vi "Bundle Zero PAS Values.vi"(7 "pasValuesByFilter In":refnum<k24>[](array[refnum]), 8 "error in (no error)":errorcluster, 10 "Results":T2[](array[typedef]), 11 "Filter Sequences":T1[](array[typedef])) -> (0 "error out":errorcluster, 1 "pasValuesByFilter Out":refnum<k24>[](array[refnum]), 4 "Filter Sequences Out":T1[](array[typedef]))   [LabVIEW 2015]
uses:
  Controls/Test Info.ctl
  Controls/Filter Sequence.ctl
  C:/Distributed/CalFlex.dll
  CalFlex.dll
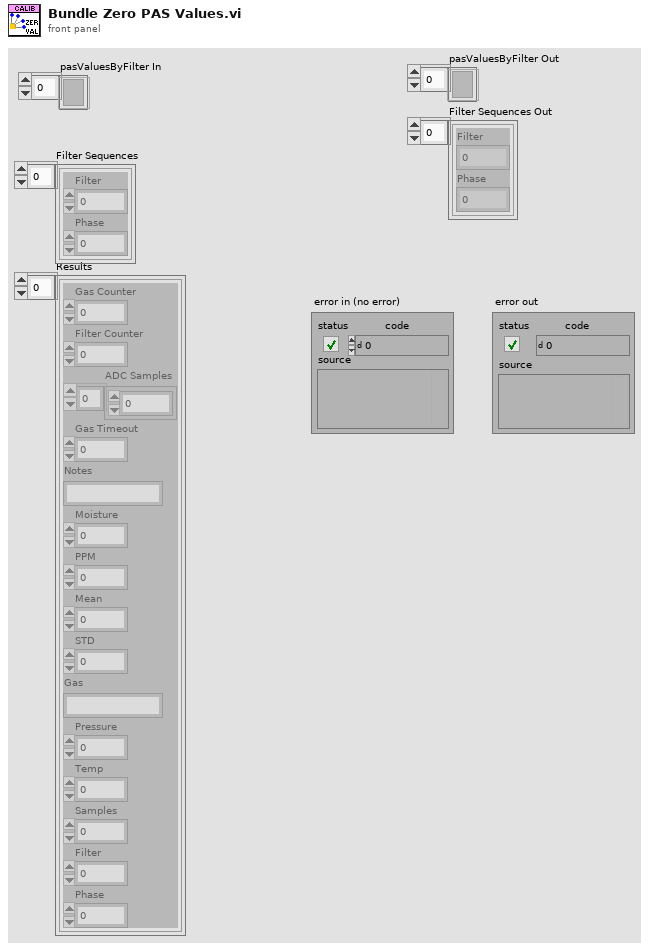
[diagram p1: front panel]
types:
  T1 = typedef "Filter Sequence.ctl" = cluster{"Filter":u8, "Phase":dbl}
  T2 = typedef "Test Info.ctl" = cluster{"Gas Counter":u16, "Filter Counter":u16, "ADC Samples":dbl[], "Gas Timeout":u16, "Notes":string, "Moisture":dbl, "PPM":dbl, "Mean":dbl, "STD":dbl, "Gas":string, "Pressure":dbl, "Temp":dbl, "Samples":u16, "Filter":u8, "Phase":dbl}
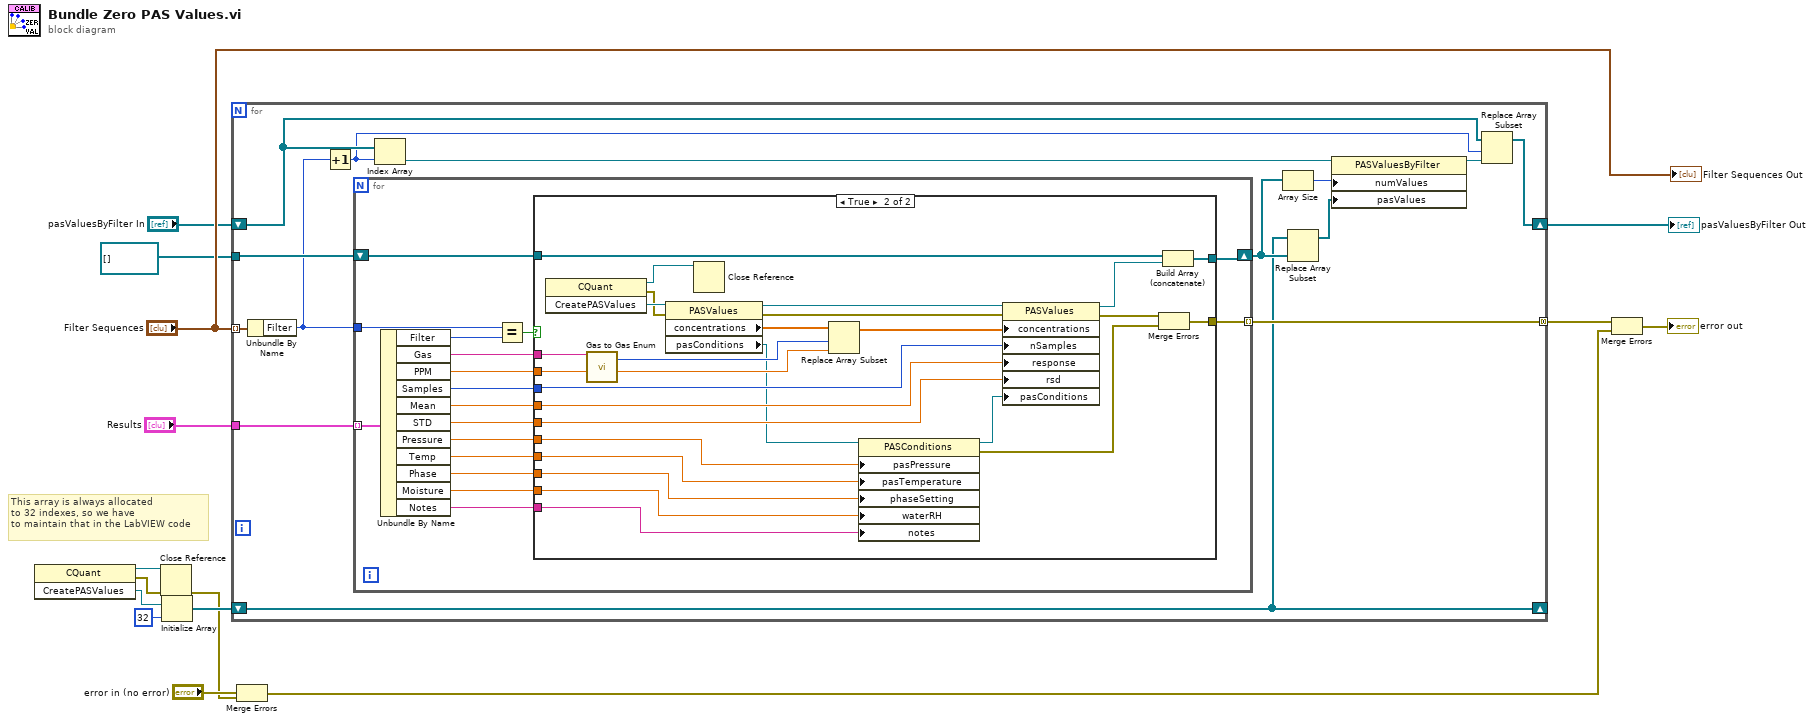
[diagram p0: block diagram]
diagram:
  # "This array is always allocated\nto 32 indexes, so we have\nto maintain that in the LabVIEW code"
  n1 = invoke class="CQuant" method="CreatePASValues"() -> (reference out=w4:refnum<k24>, error out=w5:errorcluster, "CreatePASValues"=w8:refnum<k24>)  [unwired: 3 in]
  n2 = Close Reference(reference=w4, error in (no error)=w5) -> (error out=w1:errorcluster)
  n3 = Initialize Array(w8, 32 ("dimension size")) -> (w6:refnum<k24>[])
  n4 = for {
    tunnel: "Filter Sequences" -> [w27] mode=indexing
    tunnel: "Results" -> [w29]
    tunnel: [w28] -> w15 mode=concatenating
    shift-right: [w22] -> w11
    shift-left: "pasValuesByFilter In" -> [w23]
    tunnel: refnum<k24>[] [] ("pasValues") -> [w26]
    shift-right: [w19] -> _
    shift-left: w6 -> [w19]
    n5 = Unbundle By Name(w27) -> ("Filter"=w18:u8)
    n6 = Increment(x=w18) -> (x+1=w17:u8)
    n7 = for {
      tunnel: w29 -> [w45] mode=indexing
      shift-right: [w32] -> w20
      shift-left: w26 -> [w33]
      tunnel: [w31] -> w28 mode=indexing
      tunnel: w18 -> [w30]
      n8 = Unbundle By Name(w45) -> ("Filter"=w44:u8, "Gas"=w43:string, "PPM"=w42:dbl, "Samples"=w41:u16, "Mean"=w40:dbl, "STD"=w39:dbl, "Pressure"=w38:dbl, "Temp"=w37:dbl, "Phase"=w36:dbl, "Moisture"=w35:dbl, "Notes"=w34:string)
      n9 = Equal?(x=w30, y=w44) -> (x = y?=w46:bool)
      n10 = case shown="True" w46 {
        tunnel: w43 -> [_ w70]
        tunnel: w42 -> [_ w68]
        tunnel: w41 -> [_ w55]
        tunnel: w40 -> [_ w66]
        tunnel: w39 -> [_ w65]
        tunnel: w38 -> [_ w64]
        tunnel: w37 -> [_ w63]
        tunnel: w36 -> [_ w62]
        tunnel: w35 -> [_ w48]
        tunnel: w34 -> [_ w61]
        tunnel: w33 -> [w47 w59]
        tunnel: [w47 w57] -> w32
        tunnel: [_ w56] -> w31
        frame False {
        }
        frame True {
          n11 = invoke class="CQuant" method="CreatePASValues"() -> (reference out=w49:refnum<k24>, error out=w50:errorcluster, "CreatePASValues"=w51:refnum<k24>)  [unwired: 3 in]
          n12 = call "Gas to Gas Enum.vi"("Gas"=w70) -> ("Enum"=w69:i32)  [unwired: 10 in]
          n13 = property class="PASValues"(reference=w51, error in=w50) -> (reference out=w73:refnum<k24>, error out=w72:errorcluster, "concentrations"=w71:dbl[], "pasConditions"=w52:refnum<k24>)
          n14 = Close Reference(reference=w49) -> ()  [unwired: 1 in, 1 out]
          n15 = Replace Array Subset(array=w71, new element=w68, index=w69) -> (w67:dbl[])
          n16 = property class="PASConditions"(reference=w52, "pasPressure"=w64, "pasTemperature"=w63, "phaseSetting"=w62, "waterRH"=w48, "notes"=w61) -> (reference out=w54:refnum<k24>, error out=w53:errorcluster)  [unwired: 1 in]
          n17 = property class="PASValues"(reference=w73, error in=w72, "concentrations"=w67, "nSamples"=w55, "response"=w66, "rsd"=w65, "pasConditions"=w54) -> (reference out=w58:refnum<k24>, error out=w60:errorcluster)
          n18 = Merge Errors(w60, w53) -> (w56:errorcluster)
          n19 = Build Array (concatenate)(w59, w58) -> (w57:refnum<k24>[])
        }
      }
    }
    n20 = Index Array(array=w23, index=w17) -> (element=w25:refnum<k24>)
    n21 = Array Size(array=w20) -> (size(s)=w21:i32)
    n22 = Replace Array Subset(array=w19, new element=w20) -> (w16:refnum<k24>[])  [unwired: 1 in]
    n23 = property class="PASValuesByFilter"(reference=w25, "numValues"=w21, "pasValues"=w16) -> (reference out=w24:refnum<k24>)  [unwired: 1 in, 1 out]
    n24 = Replace Array Subset(array=w23, new element=w24, index=w17) -> (w22:refnum<k24>[])
  }
  "pasValuesByFilter Out" <- w11
  n25 = Merge Errors("error in (no error)", w1) -> (w3:errorcluster)
  n26 = Merge Errors(w15, w3) -> (→"error out":errorcluster)
  "Filter Sequences Out" <- "Filter Sequences"
